vi "read block diagram numeric constant.vi"(0 "VI Ref":refnum<vi>, 7 "constant label":string, 11 "error in":errorcluster) -> (4 "dup VI Ref":refnum<vi>, 8 "constant value":i32, 15 "error out":errorcluster)   [LabVIEW 2020]
uses:
  <vilib>/Utility/traverseref.llb/TRef TravTarget.ctl
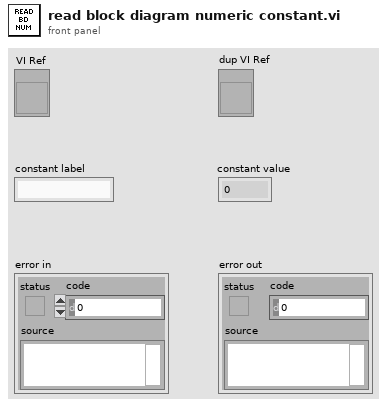
[diagram p1: front panel]
types:
  T1 = typedef "TRef TravTarget.ctl" = enum16{"FP", "BD", "Other"}
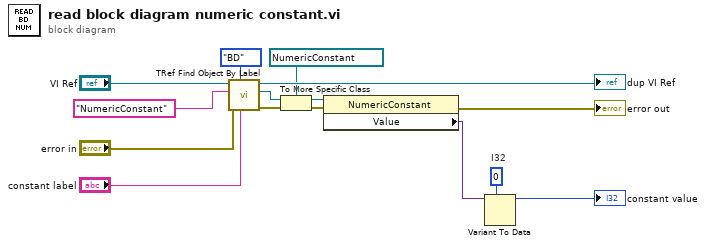
[diagram p0: block diagram]
diagram:
  w1 = 0  # I32
  n1 = call <vilib>:"TRef Find Object By Label.vi"("Label"="constant label", "Traverse Target"=TRef_TravTarget."BD", "error in (no error)"="error in", "Class Name"="NumericConstant", "VI Ref"="VI Ref") -> ("error out"=w12:errorcluster, "Found Obj Ref"=w10:refnum<vi>, "dup VI Ref"=→"dup VI Ref":refnum<vi>)  [unwired: 3 in, 1 out]
  n2 = To More Specific Class(target class=refnum<vi> refnum ("Other Refnum"), reference=w10, error in=w12) -> (specific class reference=w8:refnum<vi>, error out=w13:errorcluster)
  n3 = property class="NumericConstant"(reference=w8, error in=w13) -> (error out=→"error out":errorcluster, "Value"=w9:variant)  [unwired: 1 out]
  n4 = Variant To Data(type=w1, Variant=w9) -> (data=→"constant value":i32)  [unwired: 1 in, 1 out]
